vi "4 Axis - Set Speed.vi"(4 "error in (no error)":errorcluster, 5 "Speed":sgl, 7 "Controller Reference In":refnum<k7>) -> (0 "error out":errorcluster, 3 "Controller Reference Out":refnum<k7>)   [LabVIEW 2015]
doc: "Sets the Speed value of all 4 axis."
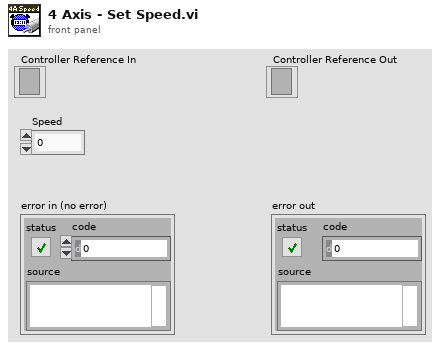
[diagram p1: front panel]
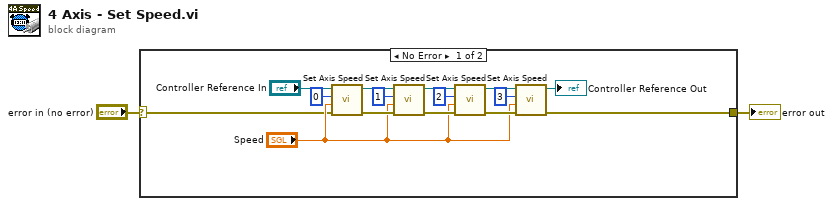
[diagram p0: block diagram]
diagram:
  n1 = case shown="No Error" "error in (no error)" {
    selector: "error in (no error)" -> [w3 w18]
    tunnel: [w4 w18] -> w2
    frame No Error {
      n2 = call "Set Axis Speed.vi"("error in (no error)"=w3, "Speed"="Speed", "Axis In"=i16 0, "Controller Reference In"="Controller Reference In") -> ("error out"=w12:errorcluster, "Controller Reference out"=w13:refnum<k7>)  [unwired: 1 in, 1 out]
      n3 = call "Set Axis Speed.vi"("error in (no error)"=w12, "Speed"="Speed", "Axis In"=i16 1, "Controller Reference In"=w13) -> ("error out"=w10:errorcluster, "Controller Reference out"=w11:refnum<k7>)  [unwired: 1 in, 1 out]
      n4 = call "Set Axis Speed.vi"("error in (no error)"=w10, "Speed"="Speed", "Axis In"=i16 2, "Controller Reference In"=w11) -> ("error out"=w8:errorcluster, "Controller Reference out"=w9:refnum<k7>)  [unwired: 1 in, 1 out]
      n5 = call "Set Axis Speed.vi"("error in (no error)"=w8, "Speed"="Speed", "Axis In"=i16 3, "Controller Reference In"=w9) -> ("error out"=w4:errorcluster, "Controller Reference out"=→"Controller Reference Out":refnum<k7>)  [unwired: 1 in, 1 out]
    }
    frame Error {
    }
  }
  "error out" <- w2
